vi "Actor Core.vi"(8 "error in":errorcluster, 11 "CS++DIMMonitor in":refnum<class "CS++DIMMonitor.lvclass">) -> (0 "error out":errorcluster, 3 "Actor out":refnum<class "Actor.lvclass">)   [LabVIEW 2013, in "CS++DIMMonitor.lvlib" / "CS++DIMMonitor.lvclass"]
doc: "(<B>Filename</B>: Actor Framework.lvlib:Actor.lvclass:Actor Core.vi)\n\nReceives messages to the actor, reacts to them, and initiates any error handling that may shut the actor down.\n\nDescendant classes may override this VI to append parallel tasks for the actor to complete while it handles messages. Overrides use the Call Parent Method node."
uses:
  CS++DIMMonitor.lvclass
  <vilib>/ActorFramework/Actor/Actor.lvclass
  <vilib>/ActorFramework/Message Enqueuer/Message Enqueuer.lvclass
  CSPP_Core/Actors/CS++PVMonitor Messages/CS++PVUpdate Msg/CS++PVUpdate Msg.lvclass
  CSPP_Core/Actors/CS++BaseActor/CS++BaseActor.lvclass/CS++BaseActor.ctl
  CS++DIMMonitor.lvclass/CS++DIMMonitor.ctl
  CSPP_Core/Actors/CS++PVMonitor/CS++PVMonitor.lvclass
  <vilib>/ActorFramework/Actor/Actor.lvclass/Actor.ctl
  <vilib>/ActorFramework/Message Enqueuer/Message Enqueuer.lvclass/Message Enqueuer.ctl
  CSPP_Core/Classes/CS++ProcessVariables/ProcessVariable/PV.lvclass
  CSPP_Core/Classes/CS++ProcessVariables/ProcessVariable/PV.lvclass/PV.ctl
  CSPP_Core/Classes/CS++ProcessVariables/ProcessVariable/Write PV URL.vi
  CSPP_Core/Classes/CS++ProcessVariables/ProcessVariable/Write Timestamp.vi
  CSPP_Core/Classes/CS++ProcessVariables/ProcessVariable/Write Data.vi
  CSPP_Core/Classes/CS++ProcessVariables/ProcessVariable/Write Error.vi
  CSPP_Core/Classes/CS++ProcessVariables/ProcessVariable/Write status.vi
  CSPP_Core/Classes/CS++ProcessVariables/ProcessVariable/Write Quality.vi
  <vilib>/ActorFramework/Message Enqueuer/Init from Existing Queue.vi
  <vilib>/ActorFramework/Message Enqueuer/Enqueue.vi
  <vilib>/ActorFramework/Message Priority Queue/Priority Enqueue.vi
  <vilib>/ActorFramework/Stop Msg/Stop Msg.lvclass
  CSPP_Core/Actors/CS++BaseActor/CS++BaseActor.lvclass
  lib.lib/DimLVEvent/LVDimInterface/LVDimInterface.lvlib
  DIMConnection/DIMConnection.lvclass
panel:
  out "no link":bool
  out "Data":variant
  out "Time Stamp":timestamp
  out "Read Error":errorcluster
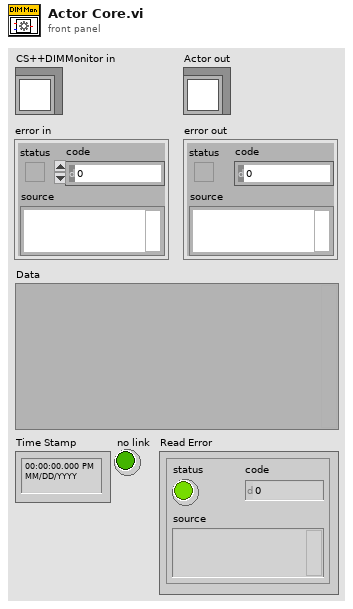
[diagram p1: front panel]
types:
  T1 = enum32{"Invalid", "Standard", "Closed", "Hidden", "Minimized", "Maximized"}
  T2 = cluster{"DIM IDs":i32[], "PV Connections":cluster{"PV URL":string, "Observers":cluster{"Enqueuer":refnum<class "Message Enqueuer.lvclass">, "CS++PVUpdate Msg":refnum<class "CS++PVUpdate Msg.lvclass">}[]}[]}
  T3 = cluster{"PV URL":string, "Observers":cluster{"Enqueuer":refnum<class "Message Enqueuer.lvclass">, "CS++PVUpdate Msg":refnum<class "CS++PVUpdate Msg.lvclass">}[]}
  T4 = cluster{"Enqueuer":refnum<class "Message Enqueuer.lvclass">, "CS++PVUpdate Msg":refnum<class "CS++PVUpdate Msg.lvclass">}[]
  T5 = cluster{"PV URL":string, "Observers":cluster{"Enqueuer":refnum<class "Message Enqueuer.lvclass">, "CS++PVUpdate Msg":refnum<class "CS++PVUpdate Msg.lvclass">}[]}[]
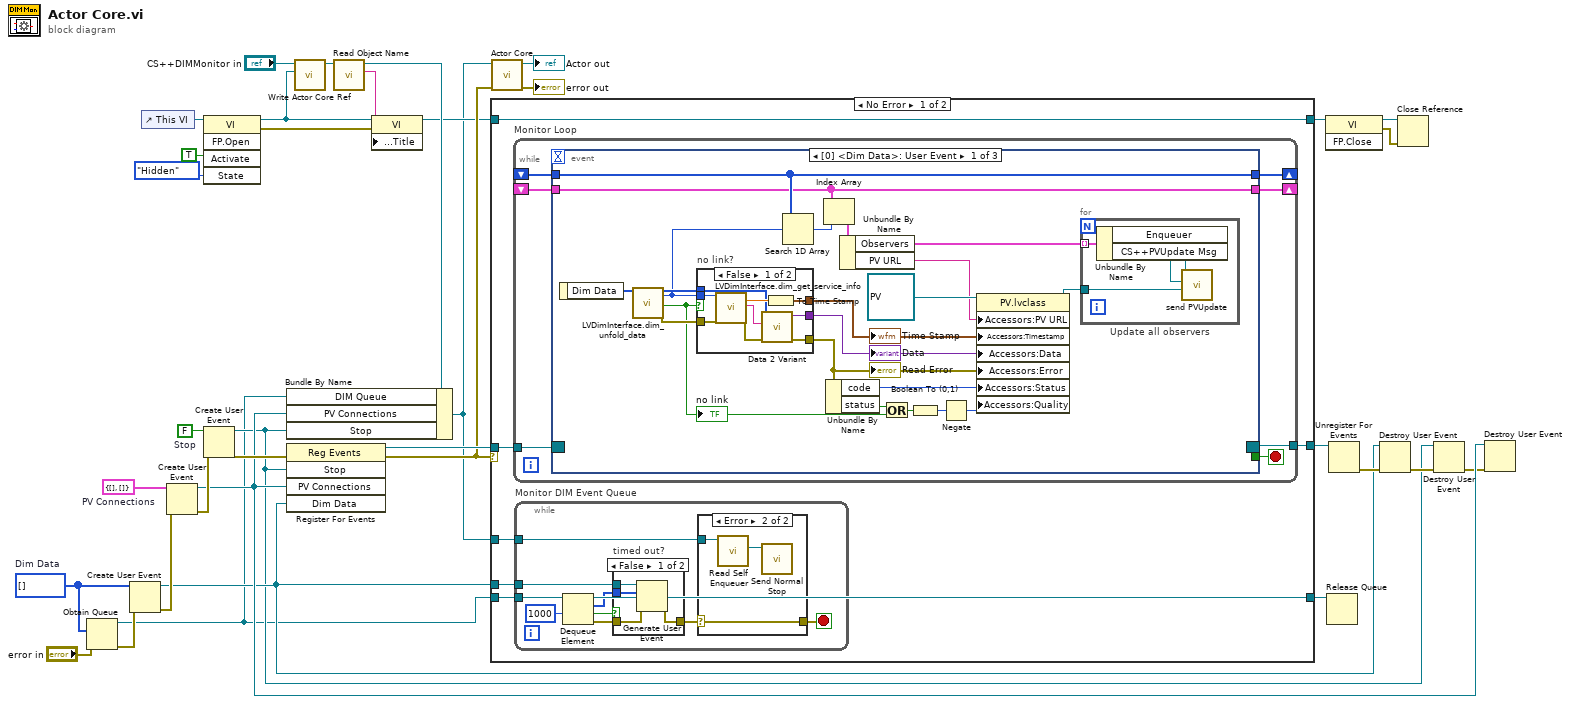
[diagram p0: block diagram]
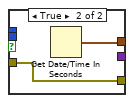
[diagram p4: hidden frame]
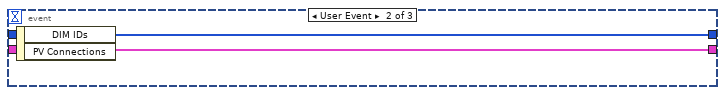
[diagram p5: hidden frame]
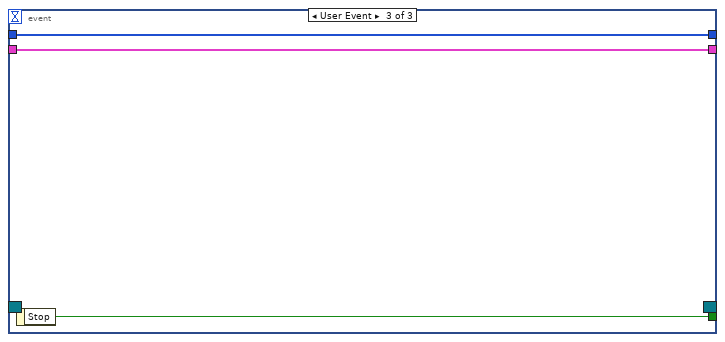
[diagram p6: hidden frame]
diagram:
  w3 = i8[] []  # Dim Data
  w11 = T2 {"DIM IDs"=[], "PV Connections"=[]}  # PV Connections
  w35 = FALSE  # Stop
  n1 = Obtain Queue(element data type=w3, error in (no error)="error in") -> (queue out=w1:refnum<queue>, error out=w9:errorcluster)  [unwired: 3 in, 1 out]
  n2 = Create User Event(user event datatype=w3, error in=w9) -> (user event=w6:refnum<user-event>, error out=w10:errorcluster)
  n3 = control-ref of="This VI"() -> (w27:refnum<vi>)
  n4 = Create User Event(user event datatype=w11, error in=w10) -> (user event=w31:refnum<user-event>, error out=w32:errorcluster)
  n5 = invoke class="VI" method="FP.Open"(reference=w27, "Activate"=TRUE ("Activate?"), "State"=T1."Hidden") -> (reference out=w21:refnum<vi>, error out=w23:errorcluster)  [unwired: 2 in, 3 out]
  n6 = Create User Event(user event datatype=w35, error in=w32) -> (user event=w5:refnum<user-event>, error out=w34:errorcluster)
  n7 = register-events(error in=w34, w5, w31, w6) -> (reference out=w33:refnum<event-registration>, error out=w28:errorcluster)  [unwired: 1 in]
  n8 = call "Write Actor Core Ref.vi"("Actor Core Ref"=w21, "CS++BaseActor in"="CS++DIMMonitor in") -> ("CS++BaseActor out"=w24:refnum<class "CS++DIMMonitor.lvclass">)  [unwired: 8 in, 1 out]
  n9 = call "Read Object Name.vi"("CS++BaseActor in"=w24) -> ("Object Name"=w22:string, "CS++BaseActor out"=w20:refnum<class "CS++DIMMonitor.lvclass">)  [unwired: 8 in, 1 out]
  n10 = Bundle By Name(cluster=w20, "DIM Queue"=w1, "PV Connections"=w31, "Stop"=w5) -> (w4:refnum<class "CS++DIMMonitor.lvclass">)
  n11 = property class="VI"(reference=w21, error in=w23, "Front Panel.Title"=w22) -> (reference out=w18:refnum<vi>)  [unwired: 1 out]
  n12 = case shown="No Error" w28 {
    tunnel: w33 -> [w41 w110]
    tunnel: [w40 w110] -> w30
    tunnel: [w39 w109] -> w19
    tunnel: w18 -> [w39 w109]
    tunnel: w1 -> [w38 w108]
    tunnel: [w38 w108] -> w12
    tunnel: w6 -> [w37 _]
    tunnel: w4 -> [w36 _]
    frame No Error {
      n13 = while "Monitor Loop" {
        tunnel: w41 -> [w66]
        tunnel: [w64] -> w40
        shift-right: [w62] -> _
        shift-left: _ -> [w63]
        shift-right: [w61] -> _
        shift-left: _ -> [w60]
        stop <- w65 stop-if-true
        n14 = event shown="[0] <Dim Data>: User Event" {
          selector: w66 -> [_ _ _]
          dyn-events: [_ _ _] -> w64
          timeout: _ -> [_ _ _]
          tunnel: [_ _ w107] -> w65
          tunnel: w63 -> [w87 _ w106]
          tunnel: [w87 w104 w106] -> w62
          tunnel: [w86 w103 w105] -> w61
          tunnel: w60 -> [w86 _ w105]
          event User Event {
            n15 = event-data() -> ("Dim Data"=w85:i8[])  [unwired: 1 in]
            n16 = call "LVDimInterface.dim_unfold_data.vi"("rawData"=w85) -> ("data"=w84:i8[], "callBackID"=w82:i32, "no link"=w67:bool, "error out"=w83:errorcluster)  [unwired: 15 in]
            "no link" <- w67
            n17 = case "no link?" shown="False" w67 {
              tunnel: w84 -> [w94 _]
              tunnel: w82 -> [w100 _]
              tunnel: w83 -> [w99 w102]
              tunnel: [w96 w102] -> w76
              tunnel: [w93 w101] -> w72
              tunnel: [w92 _] -> w71
              frame False {
                n18 = call "LVDimInterface.dim_get_service_info.vi"("callBackID"=w100, "error in (no error)"=w99) -> ("timeStamp"=w95:dbl, "typeDescriptor"=w98:string, "error out"=w97:errorcluster)  [unwired: 8 in, 7 out]
                n19 = call "Data 2 Variant.vi"("Error In"=w97, "Type Descriptor"=w98, "Data"=w94) -> ("Error Out"=w96:errorcluster, "data"=w92:variant)  [unwired: 7 in]
                n20 = To Time Stamp(1:w95) -> (0:w93:timestamp)
              }
              frame True {
                n21 = Get Date/Time In Seconds() -> (seconds since 1Jan1904=w101:timestamp)
              }
            }
            "Data" <- w71
            "Time Stamp" <- w72
            "Read Error" <- w76
            n22 = Search 1D Array(1D array=w87, element=w82) -> (index of element=w81:i32)  [unwired: 1 in]
            n23 = Index Array(array=w86, index=w81) -> (element=w80:T3)
            n24 = Unbundle By Name(w76) -> ("code"=w70:i32, "status"=w77:bool)
            n25 = Unbundle By Name(w80) -> ("Observers"=w79:T4, "PV URL"=w73:string)
            n26 = Or(x=w77, y=w67) -> (x .or. y?=w68:bool)
            n27 = Boolean To (0,1)(Boolean=w68) -> (0, 1=w78:i16)
            n28 = Negate(x=w78) -> (-x=w69:i16)
            n29 = property class="PV.lvclass"(reference=refnum<class "PV.lvclass"> refnum ("CS++ProcessVariables.lvlib:PV.lvclass"), "Accessors:PV URL"=w73, "Accessors:Timestamp"=w72, "Accessors:Data"=w71, "Accessors:Error"=w76, "Accessors:Status"=w70, "Accessors:Quality"=w69) -> (reference out=w74:refnum<class "PV.lvclass">)  [unwired: 1 in, 1 out]
            n30 = for "Update all observers" {
              tunnel: w79 -> [w91] mode=indexing
              tunnel: w74 -> [w88]
              n31 = Unbundle By Name(w91) -> ("Enqueuer"=w90:refnum<class "Message Enqueuer.lvclass">, "CS++PVUpdate Msg"=w89:refnum<class "CS++PVUpdate Msg.lvclass">)
              n32 = call "send PVUpdate.vi"("PV"=w88, "CS++PVUpdate Msg in"=w89, "Message Enqueuer in"=w90) -> ()  [unwired: 7 in, 2 out]
            }
          }
          event User Event {
            n33 = event-data() -> ("DIM IDs"=w104:i32[], "PV Connections"=w103:T5)  [unwired: 1 in]
          }
          event User Event {
            n34 = event-data() -> ("Stop"=w107:bool)  [unwired: 1 in]
          }
        }
      }
      n35 = while "Monitor DIM Event Queue" {
        tunnel: w38 -> [w49]
        tunnel: w37 -> [w48]
        tunnel: w36 -> [w44]
        stop <- w42 stop-if-true
        n36 = Dequeue Element(queue=w49, timeout in ms (-1)=1000) -> (element=w46:i8[], timed out?=w45:bool, error out=w47:errorcluster)  [unwired: 1 in, 1 out]
        n37 = case "timed out?" shown="False" w45 {
          tunnel: w48 -> [w58 _]
          tunnel: w47 -> [w57 w59]
          tunnel: w46 -> [w56 _]
          tunnel: [w55 w59] -> w43
          frame False {
            n38 = Generate User Event(user event=w58, event data cluster=w56, error in=w57) -> (error out=w55:errorcluster)  [unwired: 1 in, 1 out]
          }
          frame True {
          }
        }
        n39 = case shown="Error" w43 {
          selector: w43 -> [w51 w52]
          tunnel: w44 -> [_ w54]
          tunnel: [w51 w52] -> w42
          frame No Error {
          }
          frame Error {
            n40 = call <vilib>:"Read Self Enqueuer.vi"("Actor"=w54) -> ("Self Enqueuer"=w53:refnum<class "Message Enqueuer.lvclass">)  [unwired: 10 in]
            n41 = call <vilib>:"Send Normal Stop.vi"("Message Enqueuer"=w53) -> ()  [unwired: 10 in, 1 out]
          }
        }
      }
    }
    frame Error {
    }
  }
  n42 = call-parent "Actor Core.vi"("error in"=w28, "CS++BaseActor in"=w4) -> ("error out"=→"error out":errorcluster, "Actor out"=→"Actor out":refnum<class "Actor.lvclass">)  [unwired: 8 in]
  n43 = invoke class="VI" method="FP.Close"(reference=w19) -> (reference out=w16:refnum<vi>, error out=w17:errorcluster)  [unwired: 2 in, 1 out]
  n44 = Release Queue(queue=w12) -> ()  [unwired: 2 in, 3 out]
  n45 = Unregister For Events(event registration refnum=w30) -> (error out=w8:errorcluster)  [unwired: 1 in]
  n46 = Destroy User Event(user event=w6, error in=w8) -> (error out=w7:errorcluster)
  n47 = Close Reference(reference=w16, error in (no error)=w17) -> ()  [unwired: 1 out]
  n48 = Destroy User Event(user event=w5, error in=w7) -> (error out=w29:errorcluster)
  n49 = Destroy User Event(user event=w31, error in=w29) -> ()  [unwired: 1 out]
